vi "ex2-2.vi"() -> ()   [LabVIEW 2019]
panel:
  in  "V0":i32
  in  "q":i32
  in  "stop 2":bool
  out "Vi":dbl
  out "Ui":dbl
  in  "stop":bool
  in  "r":dbl
  in  "U0":dbl
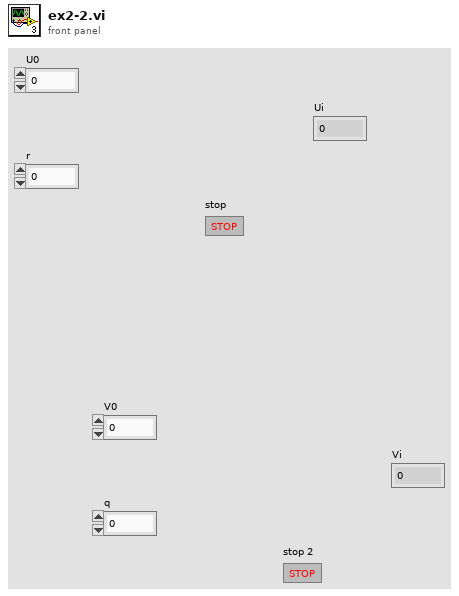
[diagram p1: front panel]
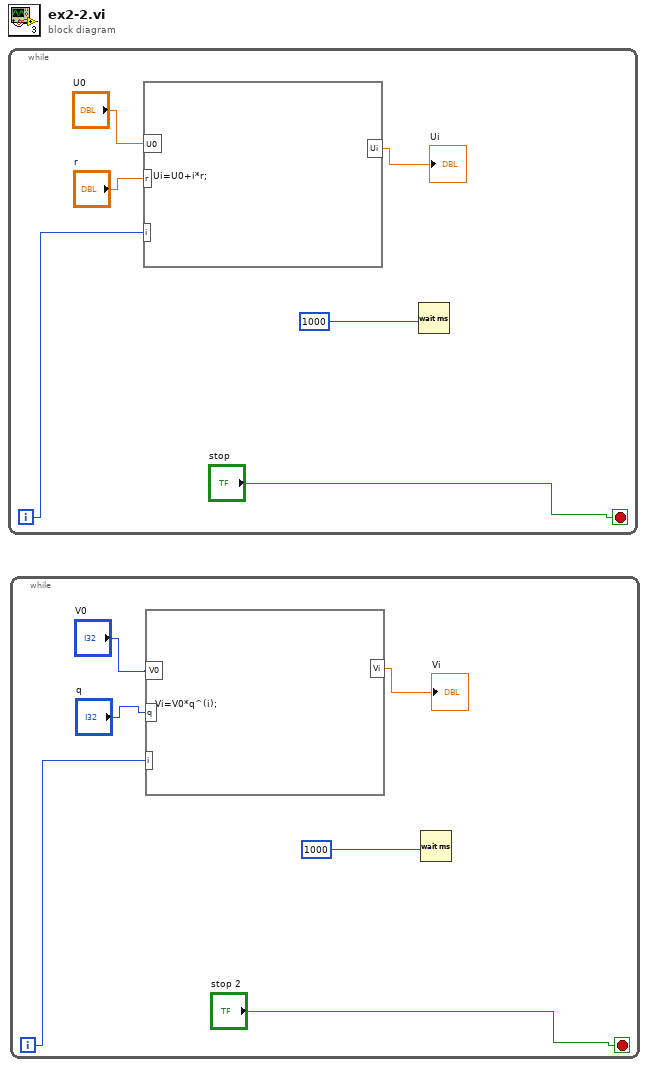
[diagram p0: block diagram]
diagram:
  n1 = while {
    i -> [w4]
    stop <- "stop" stop-if-true
    n2 = formula code="Ui=U0+i*r;"("U0"="U0", "r"="r", "i"=w4) -> ("Ui"=→"Ui":dbl)
    n3 = Wait (ms)(milliseconds to wait=1000) -> ()  [unwired: 1 out]
  }
  n4 = while {
    i -> [w12]
    stop <- "stop 2" stop-if-true
    n5 = formula code="Vi=V0*q^(i);"("i"=w12, "V0"="V0", "q"="q") -> ("Vi"=→"Vi":dbl)
    n6 = Wait (ms)(milliseconds to wait=1000) -> ()  [unwired: 1 out]
  }
